vi "initializeHeartbeat.vi"(8 "error in (no error)":errorcluster, 9 "timeout":dbl, 10 "period":dbl=1.0, 11 "tcpDevice in":refnum<class "tcpDevice.lvclass">) -> (0 "error out":errorcluster, 3 "tcpDevice out":refnum<class "tcpDevice.lvclass">)   [LabVIEW 2016, in "tcpDevice.lvclass"]
uses:
  tcpDevice.lvclass
  deviceHeartbeat/deviceHeartbeat.lvclass
  typedefs/heartbeat.ctl
  tcpDevice.lvclass/tcpDevice.ctl
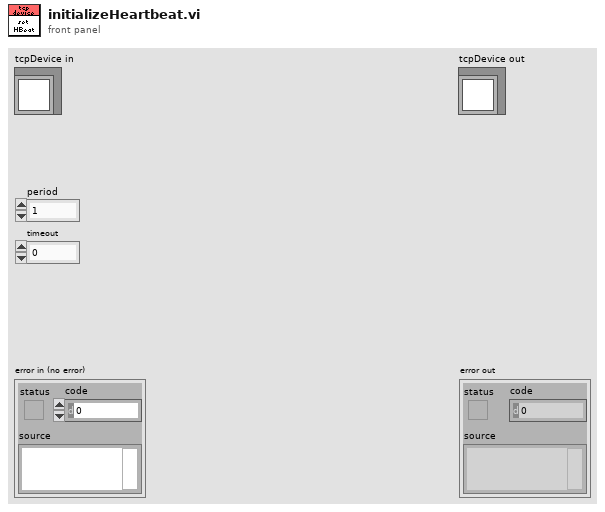
[diagram p1: front panel]
types:
  T1 = typedef "heartbeat.ctl" = cluster{"lastUpdateTime":dbl, "period":dbl, "timeout":dbl, "lastSuccesfulUpdateTime":dbl}
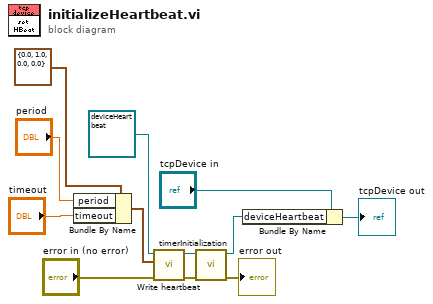
[diagram p0: block diagram]
diagram:
  n1 = Bundle By Name(cluster=T1 {"lastUpdateTime"=0.0, "period"=1.0, "timeout"=0.0, "lastSuccesfulUpdateTime"=0.0} ("heartbeat"), "period"="period", "timeout"="timeout") -> (w3:T1)
  n2 = call-dynamic "Write heartbeat.vi"("error in (no error)"="error in (no error)", "heartbeat"=w3, "deviceHeartbeat in"=refnum<class "deviceHeartbeat.lvclass"> refnum ("deviceHeartbeat.lvclass")) -> ("error out"=w7:errorcluster, "deviceHeartbeat out"=w8:refnum<class "deviceHeartbeat.lvclass">)  [unwired: 7 in]
  n3 = call "timerInitialization.vi"("error in (no error)"=w7, "deviceHeartbeat in"=w8) -> ("error out"=→"error out":errorcluster, "deviceHeartbeat out"=w10:refnum<class "deviceHeartbeat.lvclass">)  [unwired: 8 in]
  n4 = Bundle By Name(cluster="tcpDevice in", "deviceHeartbeat"=w10) -> (→"tcpDevice out":refnum<class "tcpDevice.lvclass">)
